vi "Practica_Act03.vi"() -> ()   [LabVIEW 2020]
panel:
  in  "stop":bool
  out "Voltaje":dbl
  in  "Cantidad de muestras":dbl(slide) scale=0.0..500.0
  in  "Tiempo para realizar muestras (s)":dbl(slide) scale=0.0..10.0
  out "Waveform Chart":dynamicdata(graph)
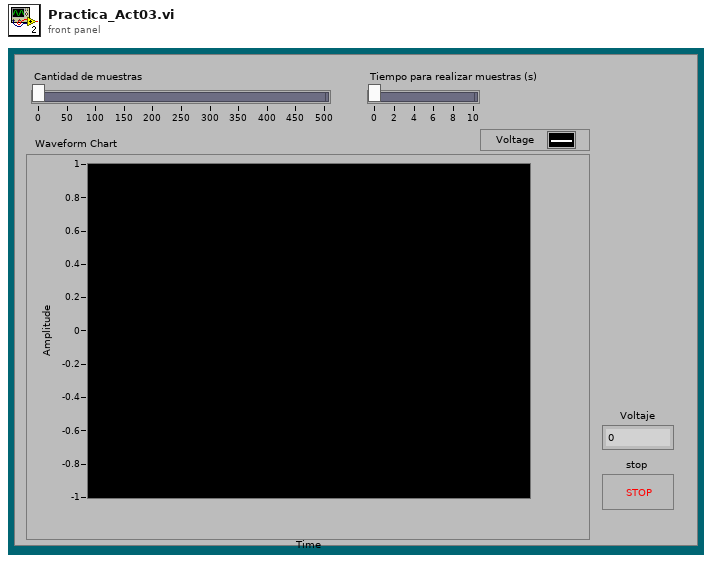
[diagram p1: front panel]
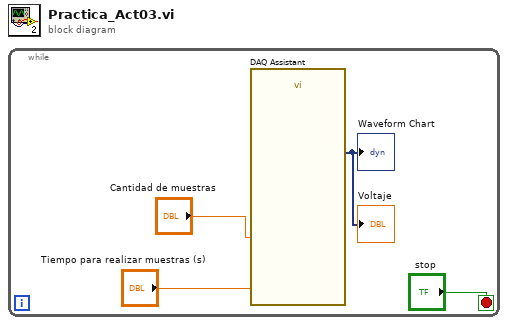
[diagram p0: block diagram]
diagram:
  n1 = while {
    stop <- "stop" stop-if-true
    n2 = call "DAQ Assistant"("number of samples"="Cantidad de muestras", "timeout (s)"="Tiempo para realizar muestras (s)") -> ("data"=→"Voltaje" →"Waveform Chart":dynamicdata)  [unwired: 15 in, 2 out]
  }
